vi "Stop Core.vi"(10 "final error code":i32, 11 "SLM_Controller in":refnum<class "SLM_Controller.lvclass">) -> (3 "SLM_Controller out":refnum<class "SLM_Controller.lvclass">)   [LabVIEW 2023, in "SLMLibrary.lvlib" / "SLM_Controller.lvlib" / "SLM_Controller.lvclass"]
doc: "(<B>Filename</B>: Actor Framework.lvlib:Actor.lvclass:Stop Core.vi)\n\nDefines what the actor does before it stops. Use the <B>final error code</B> input to determine whether the actor shut down in response to an error.\n\nBy default, this method passes the Stop message along to all auto-stop nested actors. A descendant class may override this method to define additional behavior, such as shutting down any processes the actor initiated in its override of the Actor Core method."
uses:
  SLM_Controller.lvclass
  SLM_Controller.lvclass/SLM_Controller.ctl
  <vilib>/ActorFramework/Actor/Actor.lvclass
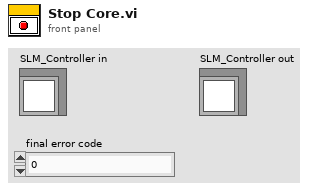
[diagram p1: front panel]
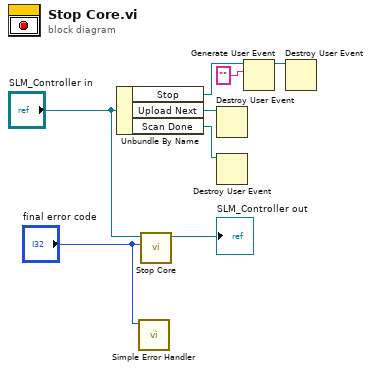
[diagram p0: block diagram]
diagram:
  n1 = Unbundle By Name("SLM_Controller in") -> ("Stop"=w6:refnum<user-event>, "Upload Next"=w3:refnum<user-event>, "Scan Done"=w2:refnum<user-event>)
  n2 = call <vilib>:"Simple Error Handler.vi"("error code (no error:0)"="final error code") -> ()  [unwired: 4 in, 5 out]
  n3 = call-parent "Stop Core.vi"("final error code"="final error code", "Actor in"="SLM_Controller in") -> ("Actor out"=→"SLM_Controller out":refnum<class "SLM_Controller.lvclass">)  [unwired: 9 in]
  n4 = Destroy User Event(user event=w3) -> ()  [unwired: 1 in, 1 out]
  n5 = Destroy User Event(user event=w2) -> ()  [unwired: 1 in, 1 out]
  n6 = Generate User Event(user event=w6, event data cluster="" ("event data")) -> (user event out=w5:refnum<user-event>)  [unwired: 2 in, 1 out]
  n7 = Destroy User Event(user event=w5) -> ()  [unwired: 1 in, 1 out]
